vi "VI Tree.vi"   [LabVIEW 2013, in "GOLPI library.lvlib"]
doc: "Contains all user VI's of the GOLPI library."
uses:
  GOLPI library.lvlib
  Get Variable/Get - Scalar - String.vi
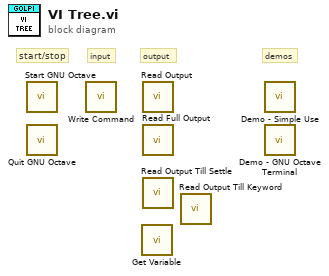
[diagram p0: block diagram]
diagram:
  # "demos"
  # "output"
  # "input"
  # "start/stop"
  n1 = call "Start GNU Octave.vi"() -> ()  [unwired: 8 in, 4 out]
  n2 = call "Quit GNU Octave.vi"() -> ()  [unwired: 10 in, 2 out]
  n3 = call "Write Command.vi"() -> ()  [unwired: 10 in, 2 out]
  n4 = call-poly "Get Variable.vi"() -> ()  [unwired: 9 in, 3 out]
  n5 = call "Read Output.vi"() -> ()  [unwired: 8 in, 4 out]
  n6 = call "Read Full Output.vi"() -> ()  [unwired: 8 in, 4 out]
  n7 = call "Read Output Till Settle.vi"() -> ()  [unwired: 8 in, 4 out]
  n8 = call "Read Output Till Keyword.vi"() -> ()  [unwired: 8 in, 4 out]
  n9 = call "Demo - Simple Use.vi"() -> ()  [unwired: 12 in]
  n10 = call "Demo - GNU Octave Terminal.vi"() -> ()  [unwired: 12 in]
